vi "Initialize With Options.vi"(7 "option string":string, 8 "error in (no error)":errorcluster {"code" format="%.0x"}, 9 "reset device (Off)":bool, 10 "id query (Off)":bool, 11 "resource string":string caption="resource name") -> (0 "error out":errorcluster {"code" format="%.0x"}, 3 "instrument handle out":refnum<k15>)   [LabVIEW 2020, in "Keysight DAQ970.lvlib"]
doc: "A string that specifies the instrument to connect to. This can \neither be a VISA resource name (also known as a VISA address) \nor an IVI session, or an IVI logical name. For PXI instruments, \na VISA resource name is of the form:\n\nPXI[bus]::[device]::INSTR\nPXI0::[bus]-[device]::INSTR\nPXI0::CHASSIS[chassis]::SLOT[slot]::INSTR\n\nFor example, the following are syntactically correct strings:\n\nPXI1::3::INSTR\nPXI0:1-3::INSTR\nPXI0::CHASSIS1::SLOT3::INSTR\n\nVISA resource names for devices connected to your computer \ncan be found using the Keysight Connection Expert. \n\nTo configure an IVI session or IVI Logical name, consult the IVI tools on your system, such as NI-MAX(Keysight devices may not appear in NI Max)."
uses:
  Keysight DAQ970.lvlib
  KtDAQ970.dll
panel:
  # "© Keysight Technologies 2020-2021"
  # "© 2000-2008 National Instruments.  All Rights Reserved."
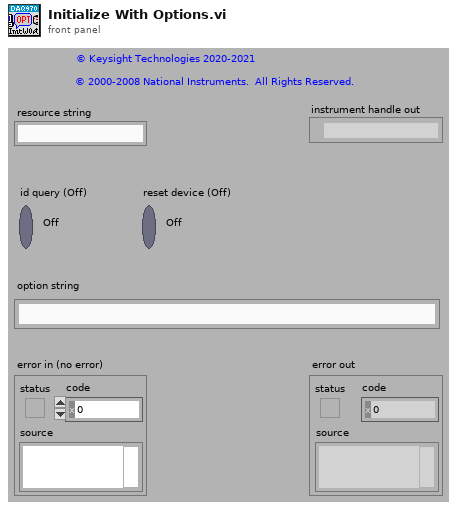
[diagram p1: front panel]
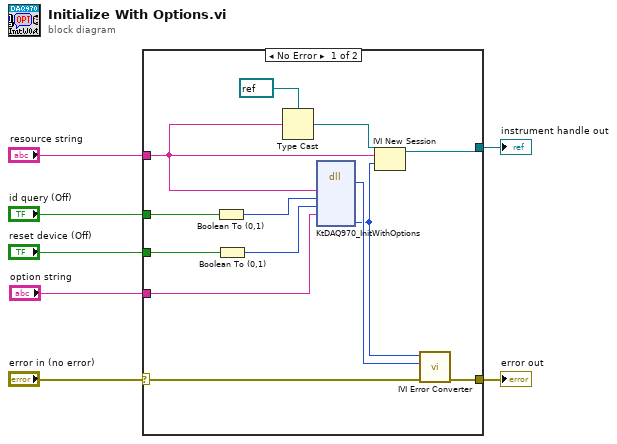
[diagram p0: block diagram]
diagram:
  n1 = case shown="No Error" "error in (no error)" {
    selector: "error in (no error)" -> [w11 w22]
    tunnel: [w10 w22] -> w6
    tunnel: "resource string" -> [w13 w21]
    tunnel: [w18 w21] -> w4
    tunnel: "id query (Off)" -> [w17 _]
    tunnel: "reset device (Off)" -> [w16 _]
    tunnel: "option string" -> [w15 _]
    frame No Error {
      n2 = Boolean To (0,1)(Boolean=w17) -> (0, 1=w20:i16)
      n3 = Boolean To (0,1)(Boolean=w16) -> (0, 1=w19:i16)
      n4 = Type Cast(type=refnum<k15> refnum ("instrument handle out"), x=w13) -> (*(type *) &x=w12:refnum<k15>)
      n5 = dll-call lib="KtDAQ970**.dll" fn="KtDAQ970_InitWithOptions" ("LabVIEW:Ivi_InitWithOptionsAndGetError")("resourceDescriptor"=w13, "idQuery"=w20, "reset"=w19, "optionString"=w15) -> ("return type"=w9:i32, "session"=w8:u32)  [unwired: 6 in, 4 out]
      n6 = IVI New Session(9:w8, 10:w13, 11:w12) -> (3:w18:refnum<k15>)
      n7 = call "IVI Error Converter.vi"("error in (no error)"=w11, "IVI error code (0)"=w9, "instrument handle"=w8) -> ("error out"=w10:errorcluster)  [unwired: 7 in, 1 out]
    }
    frame Error {
    }
  }
  "error out" <- w6
  "instrument handle out" <- w4
